vi "plugins_abort.vi"(8 "Error In":errorcluster, 10 "Plugin Index":u16, 11 "Plugins In":T1(array[cluster])) -> (0 "Error Out":errorcluster, 3 "Plugins Out":T1(array[cluster]))   [LabVIEW 2015]
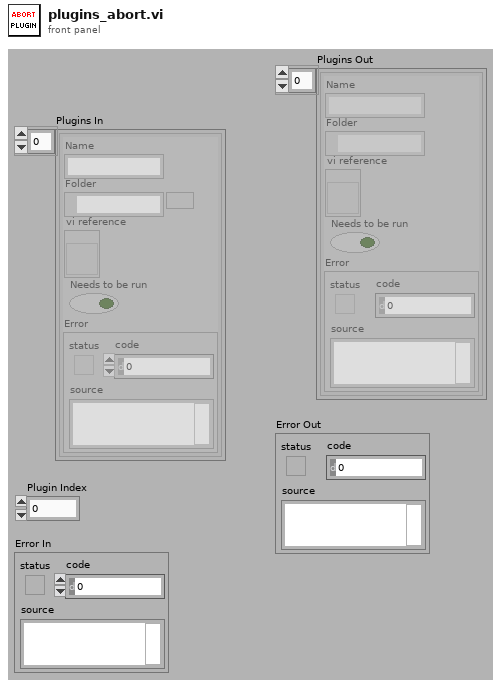
[diagram p1: front panel]
types:
  T1 = cluster{"Name":string, "Folder":path, "vi reference":refnum<vi>, "Needs to be run":bool, "Error":errorcluster}[]
  T2 = enum32{"Bad", "Idle", "Run top level", "Running"}
  T3 = cluster{"Name":string, "Folder":path, "vi reference":refnum<vi>, "Needs to be run":bool, "Error":errorcluster}
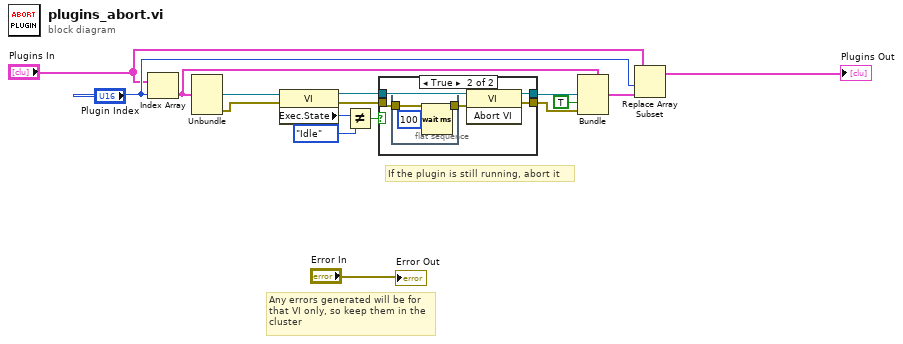
[diagram p0: block diagram]
diagram:
  # "Any errors generated will be for that VI only, so keep them in the cluster"
  # "If the plugin is still running, abort it"
  n1 = Index Array(array="Plugins In", index="Plugin Index") -> (element=w1:T3)
  n2 = Unbundle(w1) -> ("vi reference"=w11:refnum<vi>, "Error"=w12:errorcluster)  [unwired: 3 out]
  n3 = property class="VI"(reference=w11, error in=w12) -> (reference out=w7:refnum<vi>, error out=w6:errorcluster, "Exec.State"=w10:T2)
  n4 = Not Equal?(x=w10, y=T2."Idle") -> (x != y?=w8:bool)
  n5 = case shown="True" w8 {
    tunnel: w7 -> [w18 w23]
    tunnel: w6 -> [w17 w20]
    tunnel: [w17 w22] -> w4
    tunnel: [w18 w21] -> w5
    frame False {
    }
    frame True {
      n6 = flat-sequence {
        tunnel: w20 -> [w24]
        tunnel: [w24] -> w19
        frame #0 {
          n7 = Wait (ms)(milliseconds to wait=u32 100) -> ()  [unwired: 1 out]
        }
      }
      n8 = invoke class="VI" method="Abort VI"(reference=w23, error in=w19) -> (reference out=w21:refnum<vi>, error out=w22:errorcluster)  [unwired: 1 in, 1 out]
    }
  }
  n9 = Bundle(cluster=w1, "vi reference"=w5, "Needs to be run"=TRUE, "Error"=w4) -> (w2:T3)  [unwired: 2 in]
  n10 = Replace Array Subset(array="Plugins In", new element=w2, index="Plugin Index") -> (→"Plugins Out":T1)
  "Error Out" <- "Error In"
